vi "StandardMHL.vi"(8 "error in (no error)":errorcluster, 9 "Message Data":variant, 10 "Message":string, 11 "JQMHModule in":refnum<class "RQMHModule.lvclass">) -> (0 "error out":errorcluster, 3 "JQMHModule out":refnum<class "RQMHModule.lvclass">)   [LabVIEW 2024, in "RQMHModule.lvclass"]
uses:
  RQMHModule.lvclass
  RQMHModule.lvclass/RQMHModule.ctl
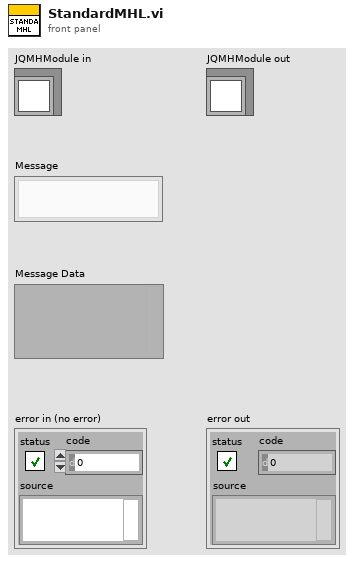
[diagram p1: front panel]
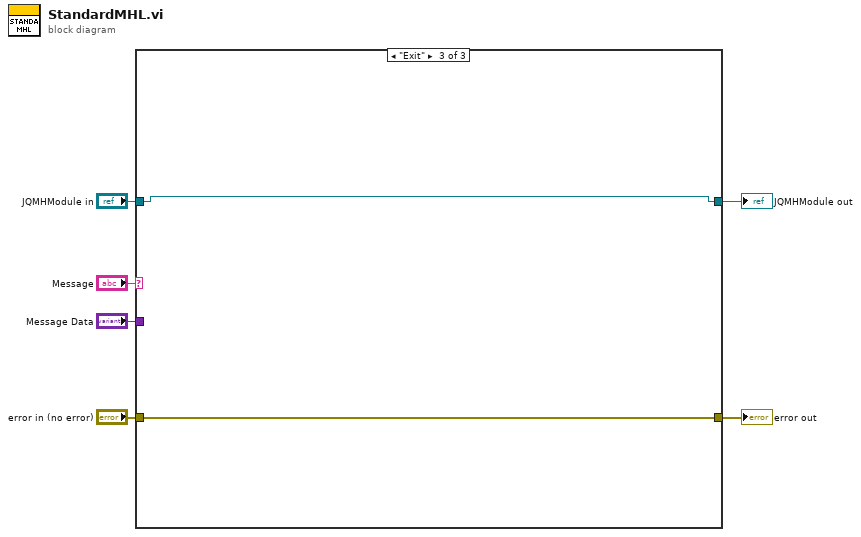
[diagram p0: block diagram]
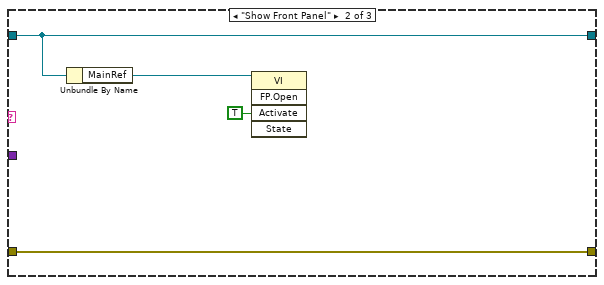
[diagram p3: hidden frame]
diagram:
  n1 = case shown="\"Exit\"" "Message" {
    tunnel: "Message Data" -> [_ _ _]
    tunnel: "JQMHModule in" -> [w8 w11 w14]
    tunnel: "error in (no error)" -> [w7 w12 w13]
    tunnel: [w7 w12 w13] -> w2
    tunnel: [w8 w11 w14] -> w1
    frame Default {
    }
    frame "Show Front Panel" {
      n2 = Unbundle By Name(w11) -> ("MainRef"=w10:refnum<vi>)
      n3 = invoke class="VI" method="FP.Open"(reference=w10, "Activate"=TRUE ("Activate?")) -> ()  [unwired: 3 in, 5 out]
    }
    frame "Exit" {
    }
  }
  "error out" <- w2
  "JQMHModule out" <- w1
